vi "Image Processing with Vision Assistant (FPGA).vi"() -> ()   [LabVIEW 2016]
uses:
  <vilib>/visionFPGA/Controls/IMAQ FPGA Image Size.ctl
  <vilib>/visionFPGA/Controls/IMAQ FPGA Pixel Bus u8x1.ctl
  <vilib>/rvi/Emulation/niFpgaGetClockAttributes.vi
  <vilib>/rvi/Emulation/niFpgaSctlEmulationGetInTimedLoop.vi
  <vilib>/rvi/Emulation/niFpgaEmulationReportErrorSimple.vi
  <vilib>/rvi/DataTransferAndStorage/Container/Common/niFpgaContainerGetUniqueNameForEmu.vi
  <vilib>/rvi/DataTransferAndStorage/Container/Common/niFpgaContainerSetEmuInfo.vi
  <vilib>/rvi/eio/common/nirviEmuReportErrorAndStop.vi
  <vilib>/visionFPGA/Basics/FIFO to Pixel Bus/IMAQ FPGA FIFO to Pixel Bus RGB32x1.vi
  <vilib>/rvi/DataTransferAndStorage/Container/Common/niFpgaContainerExecOnDevCompGetState.vi
  <vilib>/rvi/Emulation/niFpgaEmulationIsFPGAContextNoSignature.vi
  <vilib>/rvi/Emulation/niFpgaProcessEmulError.vi
  <vilib>/rvi/errors/nirviReportUnexpectedCaseInternalError (U32).vi
  <vilib>/rvi/Memory/Memory_Emulation/niFpgaMemoryEmulationCacheClearOnFirstRun.vi
  <vilib>/rvi/Memory/Memory_Emulation/nirvimemoryEmulationManagerCache_MakeExclusive.vi
  <vilib>/rvi/Memory/Memory_Emulation/niFpgaMemoryEmulationValidateCache.vi
  <vilib>/rvi/Memory/Memory_Emulation/nirvimemoryEmulationManagerCache_InsertValue.vi
  <vilib>/Utility/error.llb/Clear Errors.vi
  <vilib>/rvi/Memory/Memory_Emulation/nirvimemoryEmulationManagerCache_ReleaseExclusive.vi
  <vilib>/rvi/Memory/Memory_Emulation/nirvimemoryEmulationManagerCache_GetValue.vi
  <vilib>/rvi/Memory/Memory_Emulation/nirvimemoryEmulationManagerCache_SetValue.vi
  <vilib>/rvi/Emulation/niFpgaSctlEmulationResourceMgr.vi
  <vilib>/visionFPGA/Basics/Pixel Bus to FIFO/IMAQ FPGA Pixel Bus to FIFO U8x1.vi
  <vilib>/rvi/Emulation/niFpgaCriticalErrorInLSC.vi
  <vilib>/rvi/LocalResourceManager/LocalResourceManager.xnode
  <vilib>/rvi/DataTransferAndStorage/Container/XNode/niFpgaContainer.xnode
  <vilib>/rvi/Memory/Memory_Emulation/niFpgaMemoryEmulationRefIn.vi
  <vilib>/visionFPGA/NI_VDM_FPGA_Basics.lvlib
panel:
  out "Boolean":bool
  out "CurColNum":i16
  out "Output Line Count 2":i16
  out "Output Line Count":i16
  out "Pixel Bus In":T1
  in  "Image Size":T2={"Width"=640, "Height"=480}
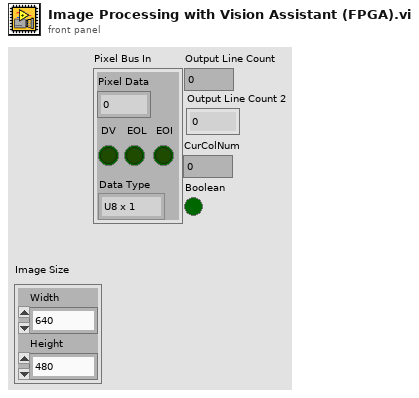
[diagram p1: front panel]
types:
  T1 = typedef "IMAQ FPGA Pixel Bus u8x1.ctl" = cluster{"Pixel Data":u8, "DV":bool, "EOL":bool, "EOI":bool, "Data Type":enum16{"U8 x 1"}}
  T2 = typedef "IMAQ FPGA Image Size.ctl" = cluster{"Width":u32, "Height":u32}
  T3 = typedef "IMAQ FPGA Pixel Bus RGB32x1.ctl" = cluster{"Pixel Data":cluster{"A":u8, "R/H":u8, "G/S":u8, "B/L":u8}, "DV":bool, "EOL":bool, "EOI":bool, "Data Type":enum16{"RGB32 x 1"}}
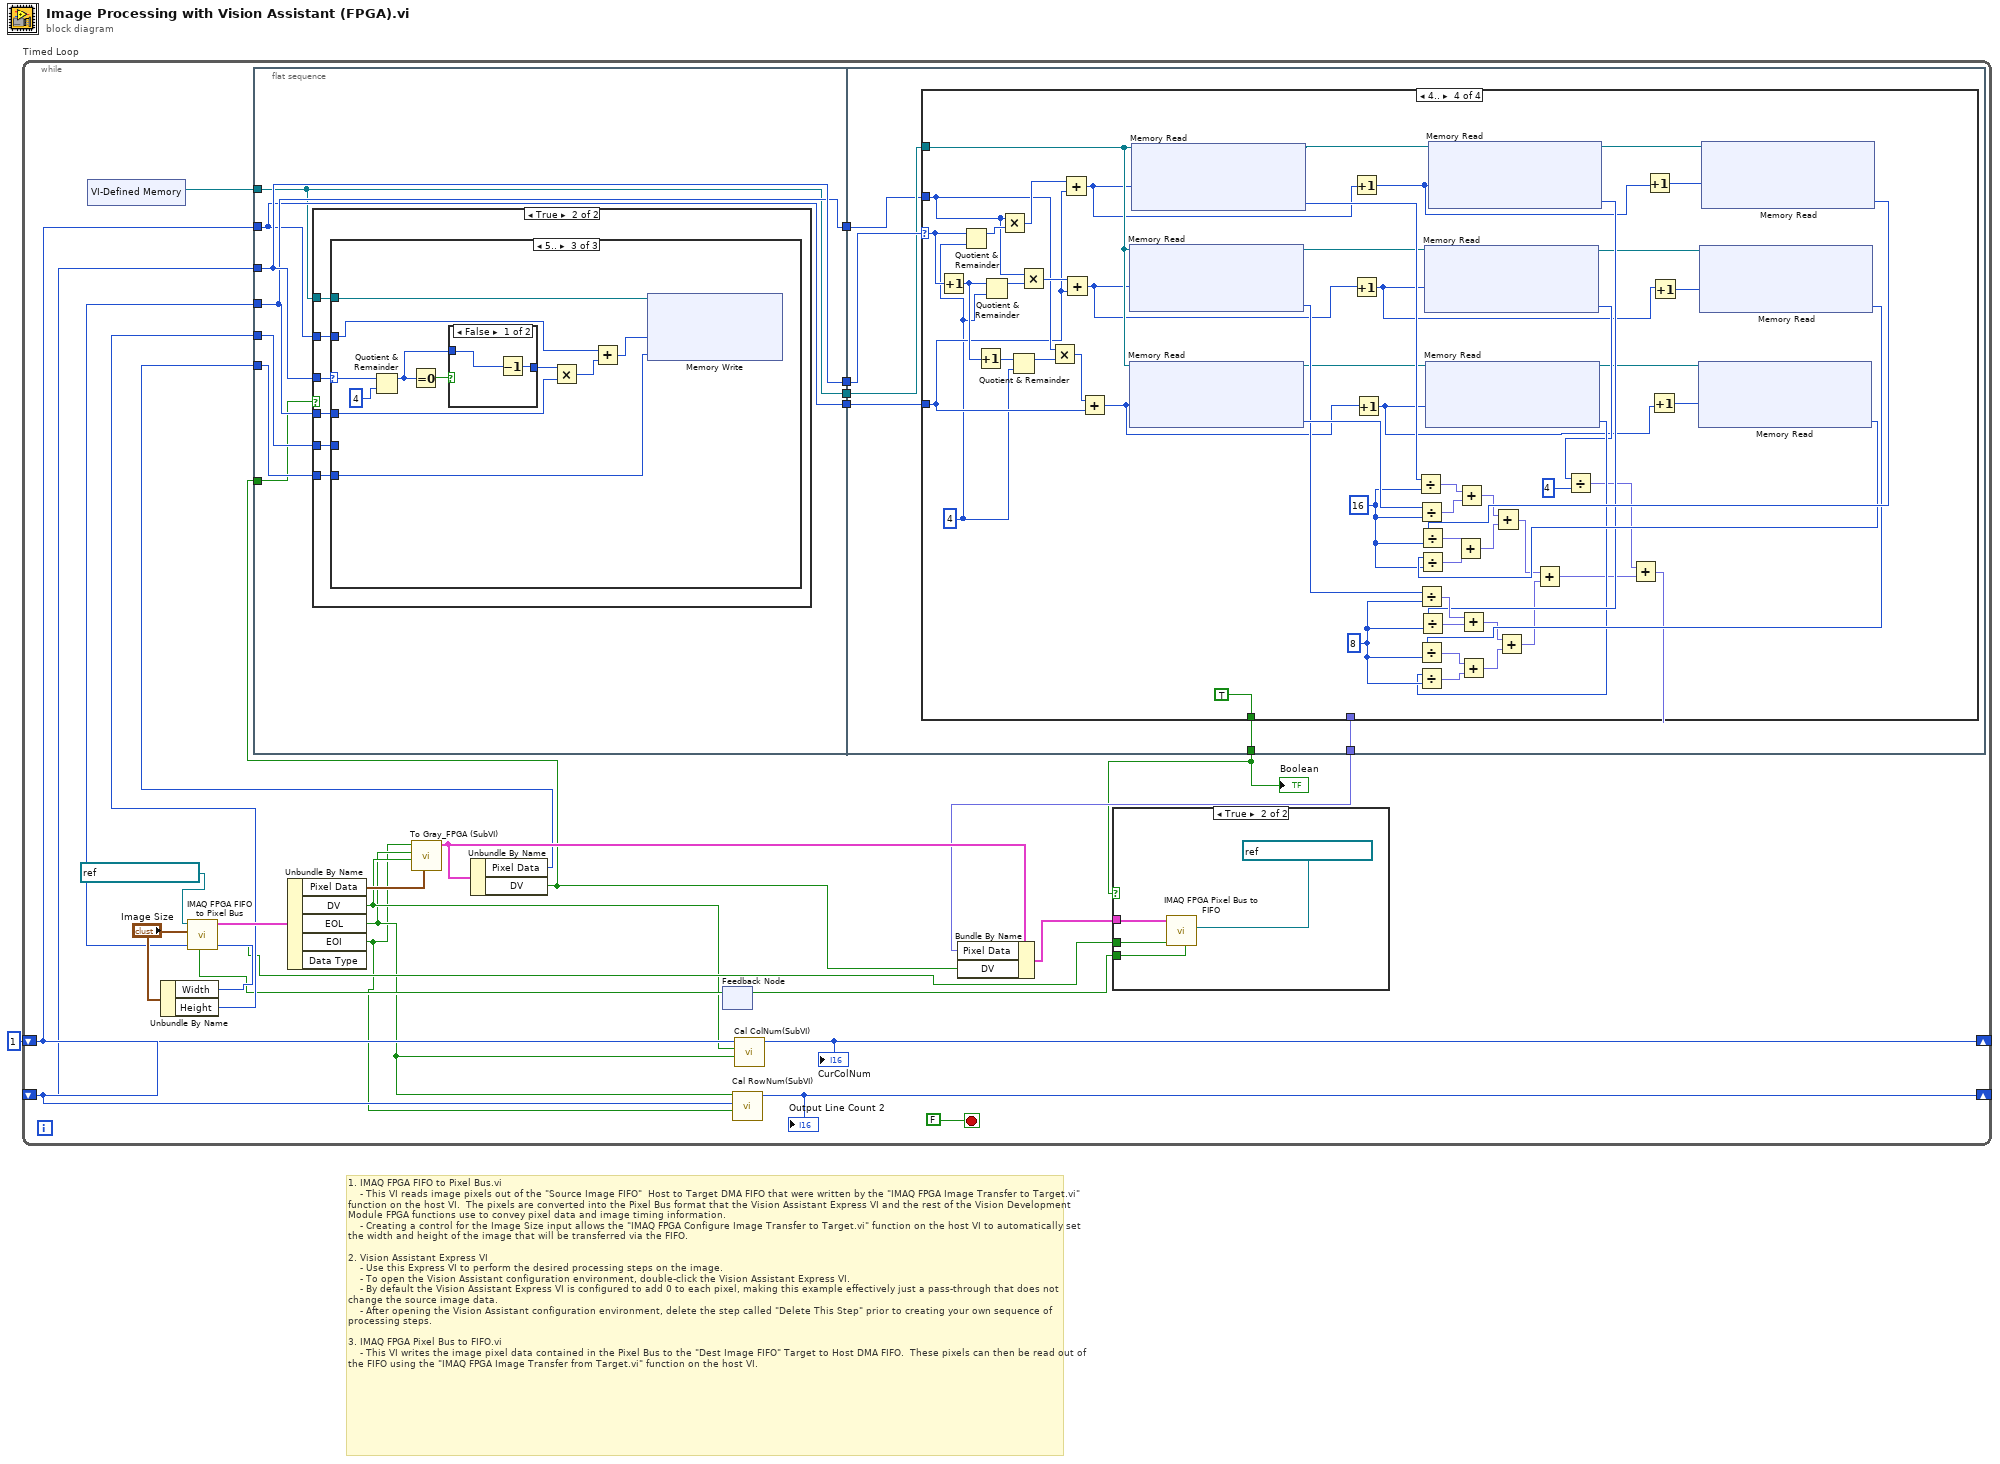
[diagram p0: block diagram]
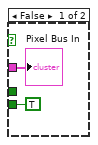
[diagram p2: hidden frame]
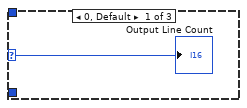
[diagram p4: hidden frame]
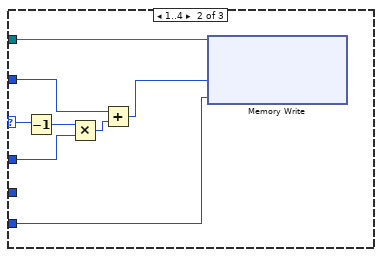
[diagram p5: hidden frame]
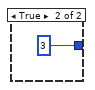
[diagram p6: hidden frame]
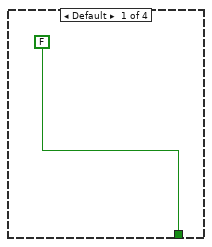
[diagram p7: hidden frame]
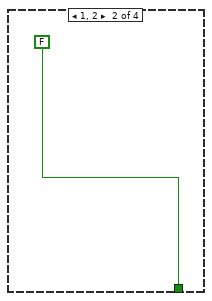
[diagram p8: hidden frame]
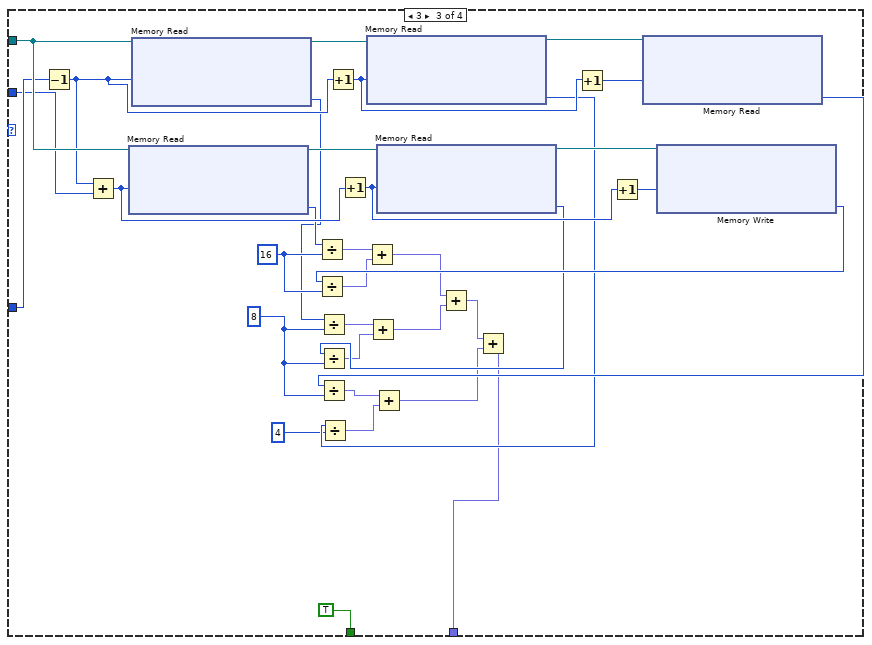
[diagram p9: hidden frame]
diagram:
  w1 = i16 1 ("Output Line Count")
  # "1. IMAQ FPGA FIFO to Pixel Bus.vi\n    - This VI reads image pixels out of the \"Source Image FIFO\"  Host to Target DMA FIFO that were written by the \"IMAQ FPGA Image Transfer to Target.vi\" function on the host VI.  The pixels are converted into the Pixel Bus format that the Vision Assistant Express VI and the rest of the Vision Development Module FPGA functions use to convey pixel data and image timing information.\n    - Creating a control for the Image Size input allows the \"IMAQ FPGA Configure Image Transfer to Target.vi\" function on the host VI to automatically set the width and height of the image that will be transferred via the FIFO.\n\n2. Vision Assistant Express VI\n    - Use this Express VI to perform the desired processing steps on the image.\n    - To open the Vision Assistant configuration environment, double-click the Vision Assistant Express VI.\n    - By default the Vision Assistant Express VI is configured to add 0 to each pixel, making this example effectively just a pass-through that does not change the source image data.\n    - After opening the Vision Assistant configuration environment, delete the step called \"Delete This Step\" prior to creating your own sequence of processing steps.\n\n3. IMAQ FPGA Pixel Bus to FIFO.vi\n    - This VI writes the image pixel data contained in the Pixel Bus to the \"Dest Image FIFO\" Target to Host DMA FIFO.  These pixels can then be read out of the FIFO using the \"IMAQ FPGA Image Transfer from Target.vi\" function on the host VI."
  n1 = while "Timed Loop" {
    shift-right: [w25] -> _
    shift-left: w1 -> [w22]
    shift-right: [w24] -> _
    shift-left: w1 -> [w20]
    stop <- FALSE stop-if-true
    n2 = xnode "VI-Defined Memory"() -> ("Memory Out"=w21:refnum<k21>)
    n3 = Unbundle By Name("Image Size") -> ("Width"=w19:u32, "Height"=w18:u32)
    n4 = flat-sequence {
      tunnel: w22 -> [w40]
      tunnel: w21 -> [w37]
      tunnel: w20 -> [w38]
      tunnel: w5 -> [w42]
      tunnel: w19 -> [w39]
      tunnel: w18 -> [w41]
      tunnel: [w40] -> w17
      tunnel: [w39] -> w16
      tunnel: [w38] -> w15
      tunnel: [w37] -> w14
      tunnel: w2 -> [w36]
      tunnel: w17 -> [w77]
      tunnel: w16 -> [w74]
      tunnel: w15 -> [w75]
      tunnel: w14 -> [w76]
      tunnel: [w73] -> w7
      tunnel: [w72] -> w6
      frame #0 {
        n5 = case shown="True" w36 {
          tunnel: w42 -> [_ w48]
          tunnel: w41 -> [_ w47]
          tunnel: w40 -> [_ w46]
          tunnel: w39 -> [_ w45]
          tunnel: w38 -> [_ w44]
          tunnel: w37 -> [_ w43]
          frame False {
          }
          frame True {
            n6 = case shown="5.." w46 {
              selector: w46 -> [w49 w56 w68]
              tunnel: w43 -> [_ w57 w60]
              tunnel: w44 -> [_ w52 w61]
              tunnel: w48 -> [_ w50 w58]
              tunnel: w45 -> [_ w54 w63]
              tunnel: w47 -> [_ _ _]
              frame 0, Default {
                "Output Line Count" <- w49
              }
              frame 1..4 {
                n7 = Decrement(x=w56) -> (x-1=w55:i16)
                n8 = Multiply(x=w55, y=w54) -> (x*y=w53:u32)
                n9 = Add(x=w52, y=w53) -> (x+y=w51:u32)
                n10 = xnode ("Memory Write")("Address"=w51, "Data"=w50, "Memory In"=w57) -> ()  [unwired: 1 out]
              }
              frame 5.. {
                n11 = Quotient & Remainder(x=w68, y=i16 4) -> (x-y*floor(x/y)=w65:i16)  [unwired: 1 out]
                n12 = Equal To 0?(x=w65) -> (x = 0?=w66:bool)
                n13 = case shown="False" w66 {
                  tunnel: w65 -> [w69 _]
                  tunnel: [w70 i16 3] -> w64
                  frame False {
                    n14 = Decrement(x=w69) -> (x-1=w70:i16)
                  }
                  frame True {
                  }
                }
                n15 = Multiply(x=w64, y=w63) -> (x*y=w62:u32)
                n16 = Add(x=w61, y=w62) -> (x+y=w59:u32)
                n17 = xnode ("Memory Write")("Address"=w59, "Data"=w58, "Memory In"=w60) -> ()  [unwired: 1 out]
              }
            }
          }
        }
      }
      frame #1 {
        n18 = case shown="4.." w77 {
          selector: w77 -> [_ _ _ w123]
          tunnel: w76 -> [_ _ w110 w139]
          tunnel: w75 -> [_ _ w108 w115]
          tunnel: w74 -> [_ _ w107 w117]
          tunnel: [_ _ w81 w136] -> w73
          tunnel: [FALSE FALSE TRUE TRUE] -> w72
          frame Default {
          }
          frame 1, 2 {
          }
          frame 3 {
            w94 = u8 8 ("y")
            w99 = u8 16 ("y")
            n19 = Decrement(x=w108) -> (x-1=w104:i16)
            n20 = Add(x=w104, y=w107) -> (x+y=w105:u32)
            n21 = xnode "Memory Read"("Address"=w105, "Memory In"=w110) -> ("Data"=w100:u8, "Memory Out"=w109:refnum<k21>)
            n22 = xnode "Memory Read"("Address"=w104, "Memory In"=w110) -> ("Data"=w95:u8, "Memory Out"=w113:refnum<k21>)
            n23 = Divide(x=w100, y=w99) -> (x/y=w97:fxp<+,8,8>)
            n24 = Divide(x=w95, y=w94) -> (x/y=w89:fxp<+,8,8>)
            n25 = Increment(x=w104) -> (x+1=w102:i16)
            n26 = Increment(x=w105) -> (x+1=w101:u32)
            n27 = xnode "Memory Read"("Address"=w102, "Memory In"=w113) -> ("Data"=w91:u8, "Memory Out"=w112:refnum<k21>)
            n28 = Divide(x=w91, y=u8 4) -> (x/y=w86:fxp<+,8,8>)
            n29 = xnode "Memory Read"("Address"=w101, "Memory In"=w109) -> ("Data"=w93:u8, "Memory Out"=w106:refnum<k21>)
            n30 = Divide(x=w93, y=w94) -> (x/y=w88:fxp<+,8,8>)
            n31 = Add(x=w89, y=w88) -> (x+y=w84:fxp<+,9,9>)
            n32 = Increment(x=w102) -> (x+1=w111:i16)
            n33 = Increment(x=w101) -> (x+1=w103:u32)
            n34 = xnode "Memory Read"("Address"=w111, "Memory In"=w112) -> ("Data"=w92:u8)  [unwired: 1 out]
            n35 = Divide(x=w92, y=w94) -> (x/y=w87:fxp<+,8,8>)
            n36 = Add(x=w87, y=w86) -> (x+y=w82:fxp<+,9,9>)
            n37 = xnode "Memory Write"("Address"=w103, "Memory In"=w106) -> ("Data"=w98:u8)  [unwired: 1 out]
            n38 = Divide(x=w98, y=w99) -> (x/y=w96:fxp<+,8,8>)
            n39 = Add(x=w97, y=w96) -> (x+y=w85:fxp<+,9,9>)
            n40 = Add(x=w85, y=w84) -> (x+y=w83:fxp<+,10,10>)
            n41 = Add(x=w83, y=w82) -> (x+y=w81:fxp<+,11,11>)
          }
          frame 4.. {
            w114 = u32 4 ("y")
            w158 = u8 8 ("y")
            w161 = u8 16 ("y")
            n42 = Increment(x=w123) -> (x+1=w121:i16)
            n43 = Quotient & Remainder(x=w123, y=w114) -> (x-y*floor(x/y)=w134:u32)  [unwired: 1 out]
            n44 = Increment(x=w121) -> (x+1=w120:i16)
            n45 = Quotient & Remainder(x=w121, y=w114) -> (x-y*floor(x/y)=w119:u32)  [unwired: 1 out]
            n46 = Multiply(x=w117, y=w134) -> (x*y=w133:u32)
            n47 = Quotient & Remainder(x=w120, y=w114) -> (x-y*floor(x/y)=w118:u32)  [unwired: 1 out]
            n48 = Multiply(x=w117, y=w119) -> (x*y=w122:u32)
            n49 = Multiply(x=w117, y=w118) -> (x*y=w116:u32)
            n50 = Add(x=w133, y=w115) -> (x+y=w130:u32)
            n51 = Add(x=w122, y=w115) -> (x+y=w127:u32)
            n52 = Add(x=w116, y=w115) -> (x+y=w126:u32)
            n53 = xnode "Memory Read"("Address"=w127, "Memory In"=w139) -> ("Data"=w157:u8, "Memory Out"=w141:refnum<k21>)
            n54 = xnode "Memory Read"("Address"=w126, "Memory In"=w139) -> ("Data"=w170:u8, "Memory Out"=w138:refnum<k21>)
            n55 = xnode "Memory Read"("Address"=w130, "Memory In"=w139) -> ("Data"=w171:u8, "Memory Out"=w143:refnum<k21>)
            n56 = Increment(x=w130) -> (x+1=w131:u32)
            n57 = Increment(x=w127) -> (x+1=w128:u32)
            n58 = Increment(x=w126) -> (x+1=w124:u32)
            n59 = Divide(x=w171, y=w161) -> (x/y=w169:fxp<+,8,8>)
            n60 = Divide(x=w170, y=w161) -> (x/y=w168:fxp<+,8,8>)
            n61 = Divide(x=w157, y=w158) -> (x/y=w160:fxp<+,8,8>)
            n62 = xnode "Memory Read"("Address"=w128, "Memory In"=w141) -> ("Data"=w153:u8, "Memory Out"=w140:refnum<k21>)
            n63 = xnode "Memory Read"("Address"=w124, "Memory In"=w138) -> ("Data"=w154:u8, "Memory Out"=w137:refnum<k21>)
            n64 = Divide(x=w154, y=w158) -> (x/y=w162:fxp<+,8,8>)
            n65 = xnode "Memory Read"("Address"=w131, "Memory In"=w143) -> ("Data"=w156:u8, "Memory Out"=w142:refnum<k21>)
            n66 = Divide(x=w156, y=w158) -> (x/y=w159:fxp<+,8,8>)
            n67 = Add(x=w169, y=w168) -> (x+y=w147:fxp<+,9,9>)
            n68 = Add(x=w160, y=w159) -> (x+y=w145:fxp<+,9,9>)
            n69 = Divide(x=w153, y=u8 4) -> (x/y=w149:fxp<+,8,8>)
            n70 = Increment(x=w131) -> (x+1=w132:u32)
            n71 = Increment(x=w124) -> (x+1=w125:u32)
            n72 = Increment(x=w128) -> (x+1=w129:u32)
            n73 = xnode "Memory Read"("Address"=w125, "Memory In"=w137) -> ("Data"=w164:u8)  [unwired: 1 out]
            n74 = Divide(x=w164, y=w161) -> (x/y=w166:fxp<+,8,8>)
            n75 = xnode "Memory Read"("Address"=w129, "Memory In"=w140) -> ("Data"=w155:u8)  [unwired: 1 out]
            n76 = Divide(x=w155, y=w158) -> (x/y=w163:fxp<+,8,8>)
            n77 = Add(x=w163, y=w162) -> (x+y=w144:fxp<+,9,9>)
            n78 = Add(x=w145, y=w144) -> (x+y=w150:fxp<+,10,10>)
            n79 = xnode "Memory Read"("Address"=w132, "Memory In"=w142) -> ("Data"=w165:u8)  [unwired: 1 out]
            n80 = Divide(x=w165, y=w161) -> (x/y=w167:fxp<+,8,8>)
            n81 = Add(x=w167, y=w166) -> (x+y=w146:fxp<+,9,9>)
            n82 = Add(x=w147, y=w146) -> (x+y=w151:fxp<+,10,10>)
            n83 = Add(x=w151, y=w150) -> (x+y=w148:fxp<+,11,11>)
            n84 = Add(x=w149, y=w148) -> (x+y=w136:fxp<+,12,12>)
          }
        }
      }
    }
    n85 = feedback #1() -> (w9:bool)  [unwired: 1 in]
    n86 = call-poly <vilib>:"IMAQ FPGA FIFO to Pixel Bus.vi"("Ready For Output"=w9, "Image Size"="Image Size", "Source Image FIFO"=refnum<k21> "32it Source FIFO") -> ("Output Valid"=w11:bool, "Pixel Bus Out"=w28:T3)  [unwired: 6 in, 1 out]
    n87 = Unbundle By Name(w28) -> ("Pixel Data"=w26:cluster{"A":u8, "R/H":u8, "G/S":u8, "B/L":u8}, "DV"=w8:bool, "EOL"=w4:bool, "EOI"=w3:bool)  [unwired: 1 out]
    n88 = call "To Gray_FPGA (SubVI).vi"("Pixel Data"=w26, "DV"=w8, "EOL"=w4, "EOI"=w3) -> ("Pixel Bus In"=w23:T1)  [unwired: 7 in]
    n89 = Unbundle By Name(w23) -> ("Pixel Data"=w5:u8, "DV"=w2:bool)
    n90 = call "Cal RowNum(SubVI).vi"("EOI"=w3, "Last Line Count"=w22, "EOL"=w4) -> ("Output Line Count"=w25:i16)  [unwired: 8 in]
    "Output Line Count 2" <- w25
    n91 = call "Cal ColNum(SubVI).vi"("EOL"=w4, "DV"=w8, "PreColNum"=w20) -> ("CurColNum"=w24:i16)  [unwired: 8 in]
    "CurColNum" <- w24
    n92 = Bundle By Name(cluster=w23, "Pixel Data"=w7, "DV"=w2) -> (w12:T1)
    n93 = case shown="True" w6 {
      tunnel: w12 -> [w31 w35]
      tunnel: w11 -> [_ w34]
      tunnel: [TRUE ("Ready for Input") w33] -> w10
      frame False {
        "Pixel Bus In" <- w31
      }
      frame True {
        n94 = call-poly <vilib>:"IMAQ FPGA Pixel Bus to FIFO.vi"("Input Valid"=w34, "Destination Image FIFO"=refnum<k21> "Dest 8bit FIFO Out", "Pixel Bus In"=w35) -> ("Ready for Input"=w33:bool)  [unwired: 8 in]
      }
    }
    n95 = feedback-in #1(w10) -> ()
    "Boolean" <- w6
  }
